vi "_RT_CtrlLoop_D999 Get_AO_Value.vi"() -> ()   [LabVIEW 2018]
uses:
  PublicSubVI/Ctl/_ctl_RT_D999_Settings.ctl
panel:
  out "error out":errorcluster
  in  "error in (no error)":errorcluster
  in  "headcmd in":string
  in  "VISA resource In":refnum<visa-resource-name>
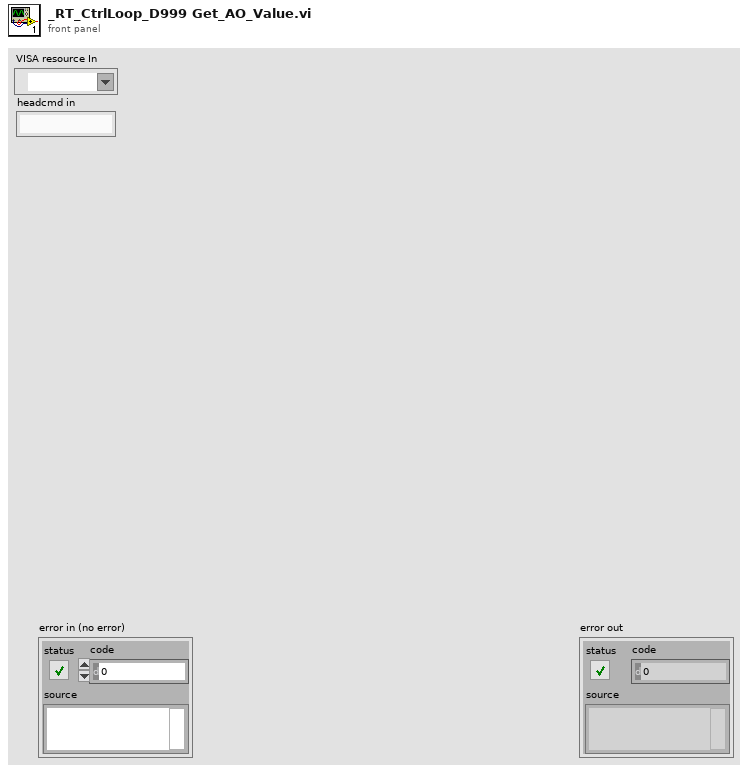
[diagram p1: front panel]
types:
  T1 = typedef "_ctl_RT_D999_Settings.ctl" = cluster{"Cmd":enum16{"None", "Init", "Write", "WriteAll", "Read", "ReadAll", "SetEnable", "SetParam", "ReadAO", "ReadSwitch", "ReportID"}, "Variant":variant}
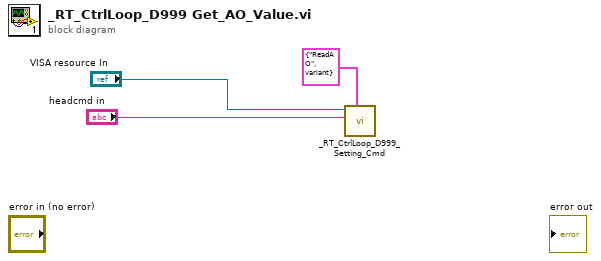
[diagram p0: block diagram]
diagram:
  n1 = call "_RT_CtrlLoop_D999_Setting_Cmd.vi"("CmdParam"=T1 {"Cmd"=enum."ReadAO", "Variant"=variant}, "VISA resource In"="headcmd in", "headcmd in"="VISA resource In") -> ()  [unwired: 4 in, 5 out]
